vi "Generate Coverage Table.vi"(8 "error in (no error)":errorcluster, 11 "Coverage Analyzer Result View In":refnum<class "Coverage Analyzer Result View.lvclass">) -> (0 "error out":errorcluster, 2 "Item Names":string[](array[string]), 3 "Coverage Analyzer Result View Out":refnum<class "Coverage Analyzer Result View.lvclass">)   [LabVIEW 2020, in "Coverage Analyzer Result View.lvclass"]
uses:
  Coverage Analyzer Result View.lvclass
  Coverage Analyzer Result View.lvclass/Coverage Analyzer Result View.ctl
  5b3a251b-490d-4765-8bc6-b6b8562e6ece.vi
  <vilib>/Comparison/Less/Less Functor/Less Functor.lvclass
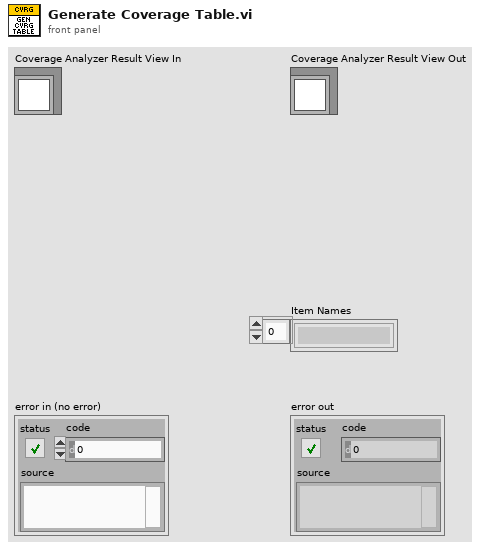
[diagram p1: front panel]
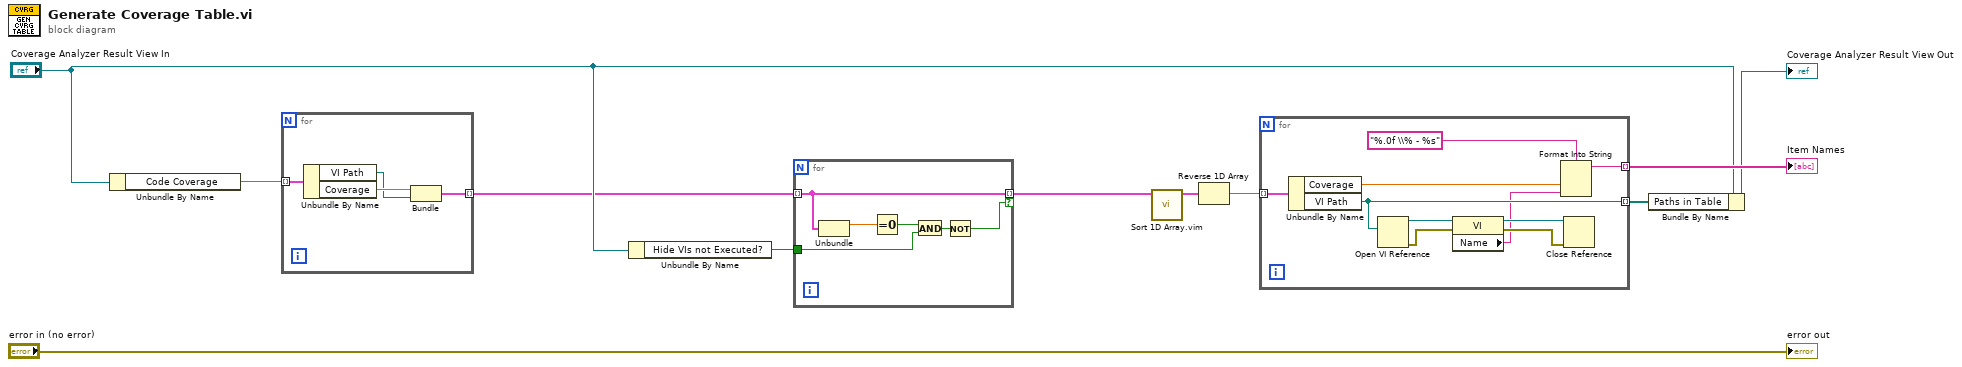
[diagram p0: block diagram]
diagram:
  n1 = Unbundle By Name("Coverage Analyzer Result View In") -> ("Code Coverage"=w6:map{path, dbl})
  n2 = for {
    tunnel: w6 -> [w15] mode=indexing
    tunnel: [w13] -> w3 mode=indexing
    n3 = Unbundle By Name(w15) -> ("VI Path"=w12:path, "Coverage"=w14:dbl)
    n4 = Bundle("Coverage"=w14, "VI Path"=w12) -> (w13:cluster{"Coverage":dbl, "VI Path":path})  [unwired: 1 in]
  }
  n5 = Unbundle By Name("Coverage Analyzer Result View In") -> ("Hide VIs not Executed?"=w1:bool)
  n6 = for {
    tunnel: [w21] -> w2 mode=indexing if=w16
    tunnel: w3 -> [w21] mode=indexing
    tunnel: w1 -> [w18]
    n7 = Unbundle(w21) -> ("Coverage"=w20:dbl)  [unwired: 1 out]
    n8 = Equal To 0?(x=w20) -> (x = 0?=w19:bool)
    n9 = And(x=w19, y=w18) -> (x .and. y?=w17:bool)
    n10 = Not(x=w17) -> (.not. x?=w16:bool)
  }
  n11 = call "Sort 1D Array.vim"("unsorted array"=w2) -> ("sorted array"=w10:cluster{"Coverage":dbl, "VI Path":path}[])  [unwired: 10 in]
  n12 = Reverse 1D Array(array=w10) -> (reversed array=w8:cluster{"Coverage":dbl, "VI Path":path}[])
  n13 = for {
    tunnel: w8 -> [w31] mode=indexing
    tunnel: [w28] -> w9 mode=indexing
    tunnel: [w23] -> w5 mode=indexing
    n14 = Unbundle By Name(w31) -> ("Coverage"=w29:dbl, "VI Path"=w23:path)
    n15 = Open VI Reference(vi path=w23) -> (vi reference=w27:refnum<vi>, error out=w26:errorcluster)  [unwired: 5 in]
    n16 = property class="VI"(reference=w27, error in=w26) -> (reference out=w25:refnum<vi>, error out=w24:errorcluster, "Name"=w22:string)
    n17 = Format Into String(format string="%.0f \\% - %s", w29, w22) -> (resulting string=w28:string)  [unwired: 2 in, 1 out]
    n18 = Close Reference(reference=w25, error in (no error)=w24) -> ()  [unwired: 1 out]
  }
  "Item Names" <- w9
  n19 = Bundle By Name(cluster="Coverage Analyzer Result View In", "Paths in Table"=w5) -> (→"Coverage Analyzer Result View Out":refnum<class "Coverage Analyzer Result View.lvclass">)
  "error out" <- "error in (no error)"
